vi "I-O Test.vi"() -> ()   [LabVIEW 2021]
uses:
  Classes/Controller/I-O/I-O.lvclass
  Classes/Controller/Controller.lvclass
panel:
  out "Compression Sensor":bool=TRUE
  out "Sensor Channel":dbl
  out "Sensor":bool=TRUE
  out "sensor pin number":i32
  out "tray sensor":bool
  out "secondary valve sensor":bool
  out "primary valve sensor":bool
  in  "Turn on secondary vacuum":bool
  in  "turn on primary vacuum":bool
  in  "secure tray":bool
  out "Valve Channel":dbl
  in  "Type":enum16{"O ring Vac", "Baseplate Vac"}(ring)
  in  "Position":i32
  in  "Region":i32
  in  "On/Off":bool
  in  "Stop":bool
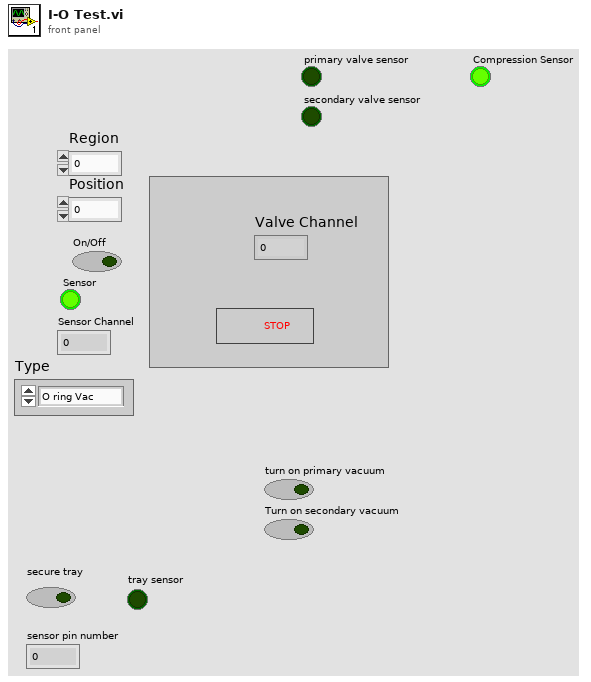
[diagram p1: front panel]
types:
  T1 = typedef "Controller.lvclass/Controllers.ctl" = cluster{"I-O.lvclass":refnum<class "I-O.lvclass">, "Gantry":refnum<k24>, "Dispenser":refnum<visa-resource-name>}
  T2 = typedef "I-O.lvclass/Pin Map.ctl" = cluster{"Region Valves":i32[], "Extra Valves":dbl[][][], "Tool Primary Valve":i32, "Tool Secondary Valve":i32, "Region Sensors":i32[], "Extra Sensors":dbl[][][], "Tool Primary Sensor":dbl, "Tool Secondary Sensor":dbl, "Compression Sensor":dbl, "5V":i32, "Dispenser Sensor":dbl}
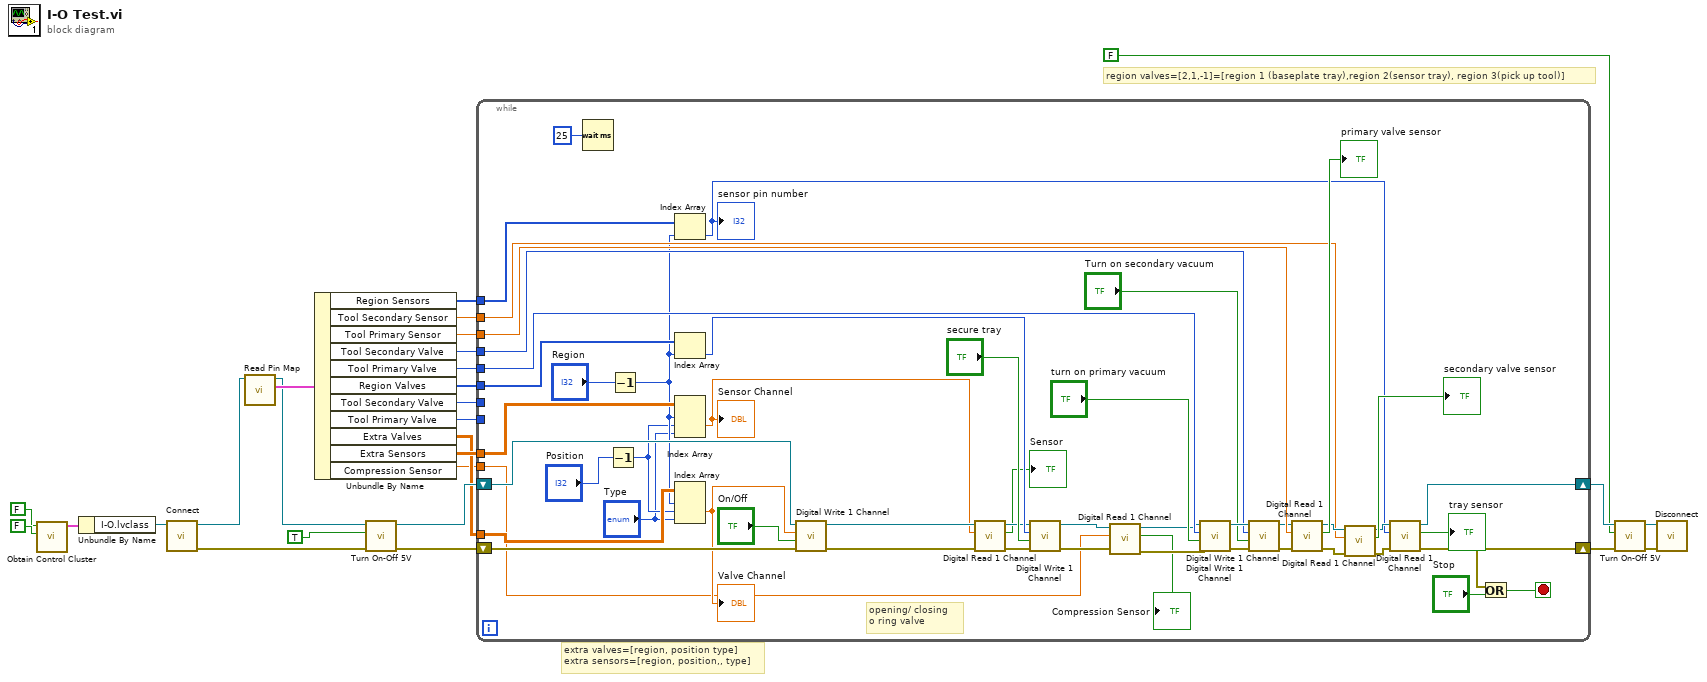
[diagram p0: block diagram]
diagram:
  # "extra valves=[region, position type]\nextra sensors=[region, position,, type]"
  # "region valves=[2,1,-1]=[region 1 (baseplate tray),region 2(sensor tray), region 3(pick up tool)]"
  n1 = call "Obtain Control Cluster.vi"("Dispense"=FALSE, "Motion"=FALSE) -> ("Control Out"=w11:T1)  [unwired: 9 in]
  n2 = Unbundle By Name(w11) -> ("I-O.lvclass"=w10:refnum<class "I-O.lvclass">)
  n3 = call-dynamic "Connect.vi"("Controller in"=w10) -> ("error out"=w18:errorcluster, "Controller out"=w20:refnum<class "I-O.lvclass">)  [unwired: 9 in]
  n4 = call-dynamic "Read Pin Map.vi"("I-O in"=w20) -> ("Pin Map 2"=w22:T2, "I-O out"=w21:refnum<class "I-O.lvclass">)  [unwired: 8 in, 1 out]
  n5 = Unbundle By Name(w22) -> ("Region Sensors"=w1:i32[], "Tool Secondary Sensor"=w2:dbl, "Tool Primary Sensor"=w3:dbl, "Tool Secondary Valve"=w4:i32, "Tool Primary Valve"=w5:i32, "Region Valves"=w6:i32[], "Tool Secondary Valve"=w8:i32, "Tool Primary Valve"=w7:i32, "Extra Valves"=w14:dbl[][][], "Extra Sensors"=w19:dbl[][][], "Compression Sensor"=w9:dbl)
  n6 = call-dynamic "Turn On-Off 5V.vi"("error in (no error)"=w18, "Value"=TRUE, "I-O in"=w21) -> ("error out"=w17:errorcluster, "I-O out"=w27:refnum<class "I-O.lvclass">)  [unwired: 7 in]
  n7 = while {
    shift-right: [w47] -> w24
    shift-left: w27 -> [w74]
    tunnel: w19 -> [w38]
    shift-right: [w49] -> w16
    shift-left: w17 -> [w73]
    tunnel: w14 -> [w39]
    tunnel: w9 -> [w29]
    tunnel: w8 -> [_]
    tunnel: w7 -> [_]
    tunnel: w6 -> [w68]
    tunnel: w5 -> [w65]
    tunnel: w4 -> [w62]
    tunnel: w3 -> [w59]
    tunnel: w2 -> [w54]
    tunnel: w1 -> [w51]
    stop <- w75 stop-if-true
    # "opening/ closing \no ring valve"
    n8 = Wait (ms)(milliseconds to wait=u32 25) -> ()  [unwired: 1 out]
    n9 = Decrement(x="Position") -> (x-1=w36:i32)
    n10 = Decrement(x="Region") -> (x-1=w37:i32)
    n11 = Index Array(array=w51, index=w37) -> (element=w46:i32)
    "sensor pin number" <- w46
    n12 = Index Array(array=w68, index=w37) -> (element=w67:i32)
    n13 = Index Array(array=w38, index (dim 0)=w37, index (dim 1)=w36, index (dim 2)="Type") -> (element=w34:dbl)
    "Sensor Channel" <- w34
    n14 = Index Array(array=w39, index (dim 0)=w37, index (dim 1)=w36, index (dim 2)="Type") -> (element=w69:dbl)
    "Valve Channel" <- w69
    n15 = call-dynamic "Digital Write 1 Channel.vi"("error constant"=w73, "Value"="On/Off", "Channel"=w69, "I-O.lvclass"=w74) -> ("error IO"=w43:errorcluster, "I-O.lvclass 2"=w44:refnum<class "I-O.lvclass">)  [unwired: 6 in]
    n16 = call-dynamic "Digital Read 1 Channel.vi"("error in (no error)"=w43, "Read"=w34, "I-O in"=w44) -> ("error out"=w42:errorcluster, "Value"=→"Sensor":bool, "I-O out"=w41:refnum<class "I-O.lvclass">)  [unwired: 6 in]
    n17 = call-dynamic "Digital Write 1 Channel.vi"("error constant"=w42, "Value"="secure tray", "Channel"=w67, "I-O.lvclass"=w41) -> ("error IO"=w33:errorcluster, "I-O.lvclass 2"=w32:refnum<class "I-O.lvclass">)  [unwired: 6 in]
    n18 = call-dynamic "Digital Read 1 Channel.vi"("error in (no error)"=w33, "Read"=w29, "I-O in"=w32) -> ("error out"=w30:errorcluster, "Value"=→"Compression Sensor":bool, "I-O out"=w31:refnum<class "I-O.lvclass">)  [unwired: 6 in]
    n19 = call-dynamic "Digital Write 1 Channel.vi"("error constant"=w30, "Value"="turn on primary vacuum", "Channel"=w65, "I-O.lvclass"=w31) -> ("error IO"=w60:errorcluster, "I-O.lvclass 2"=w63:refnum<class "I-O.lvclass">)  [unwired: 6 in]
    n20 = call-dynamic "Digital Write 1 Channel.vi"("error constant"=w60, "Value"="Turn on secondary vacuum", "Channel"=w62, "I-O.lvclass"=w63) -> ("error IO"=w56:errorcluster, "I-O.lvclass 2"=w58:refnum<class "I-O.lvclass">)  [unwired: 6 in]
    n21 = call-dynamic "Digital Read 1 Channel.vi"("error in (no error)"=w56, "Read"=w59, "I-O in"=w58) -> ("error out"=w52:errorcluster, "Value"=→"primary valve sensor":bool, "I-O out"=w55:refnum<class "I-O.lvclass">)  [unwired: 6 in]
    n22 = call-dynamic "Digital Read 1 Channel.vi"("error in (no error)"=w52, "Read"=w54, "I-O in"=w55) -> ("error out"=w50:errorcluster, "Value"=→"secondary valve sensor":bool, "I-O out"=w48:refnum<class "I-O.lvclass">)  [unwired: 6 in]
    n23 = call-dynamic "Digital Read 1 Channel.vi"("error in (no error)"=w50, "Read"=w46, "I-O in"=w48) -> ("error out"=w49:errorcluster, "Value"=→"tray sensor":bool, "I-O out"=w47:refnum<class "I-O.lvclass">)  [unwired: 6 in]
    n24 = Or(x=w49, y="Stop") -> (x .or. y?=w75:bool)
  }
  n25 = call-dynamic "Turn On-Off 5V.vi"("error in (no error)"=w16, "Value"=FALSE, "I-O in"=w24) -> ("error out"=w15:errorcluster, "I-O out"=w25:refnum<class "I-O.lvclass">)  [unwired: 7 in]
  n26 = call-dynamic "Disconnect.vi"("error in (no error)"=w15, "I-O in"=w25) -> ()  [unwired: 8 in, 1 out]
